vi "Find_Potentially_Stat_Dots_In_Dot-Matrix-1.vi"(4 "[IN] Count of event \"+1\"":i32, 5 "[IN] Dot matrix with \nstatuses after searching \nof unmoving dots":i16[][](array[numeric]), 6 "[IN] Possibly\nMoving (X,Y)":dbl[][](array[numeric]), 7 "Current # frame":i32, 8 "Y2":dbl, 9 "X2":dbl, 10 "Y1":dbl, 11 "X1":dbl) -> (1 "[OUT] Count of event \"+1\" 2":i32, 3 "[OUT] Dot matrix with \nstatuses after searching \nof unmoving dots":i16[][](array[numeric]))   [LabVIEW 2013]
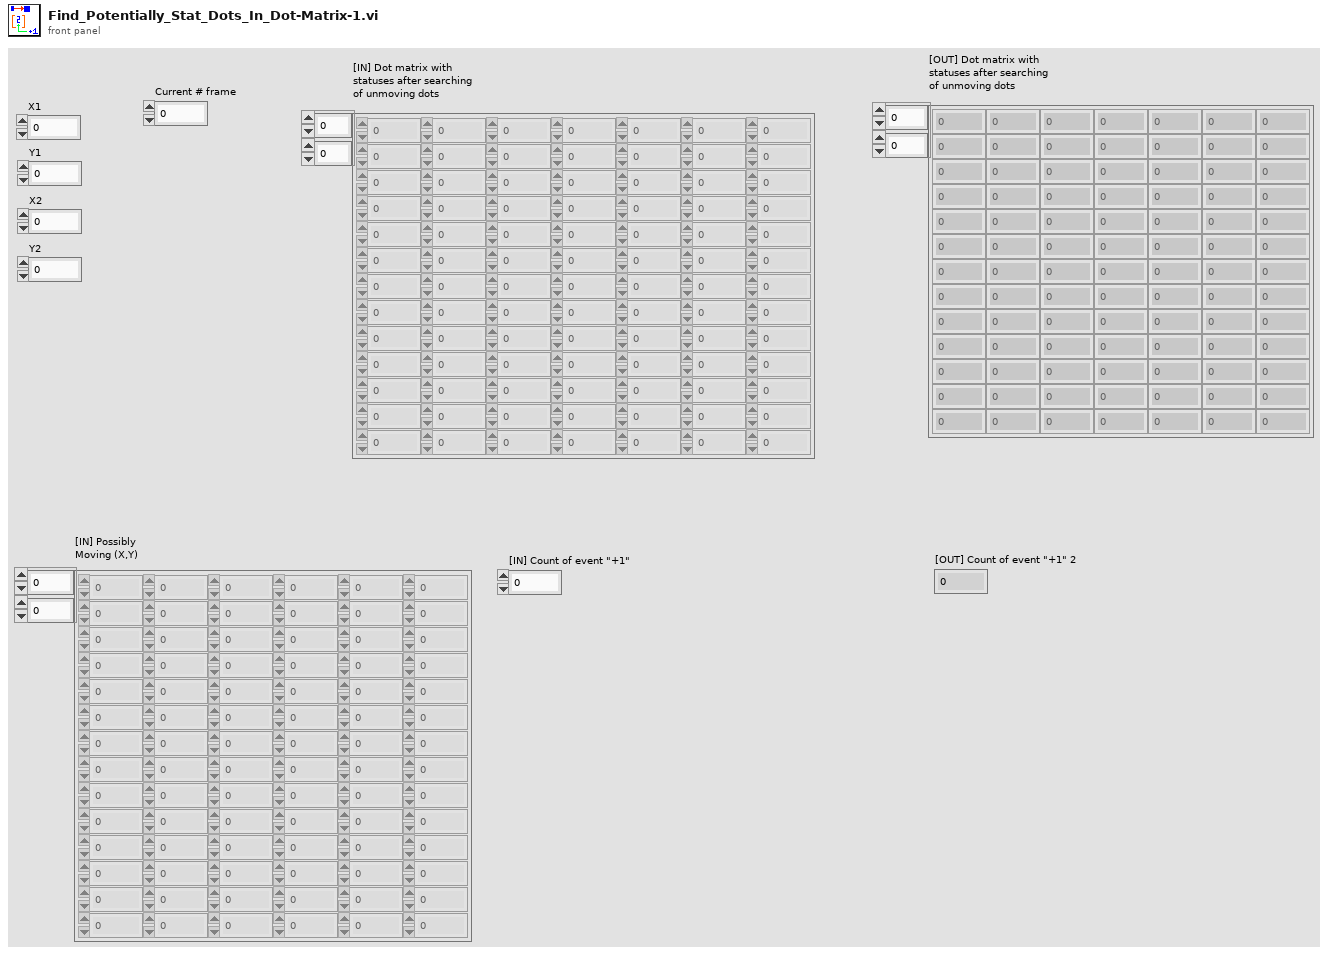
[diagram p1: front panel]
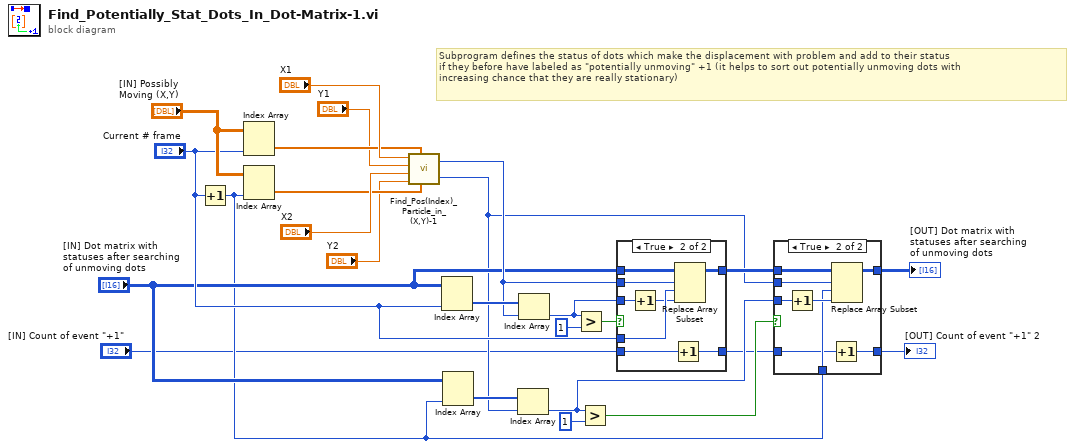
[diagram p0: block diagram]
diagram:
  # "Subprogram defines the status of dots which make the displacement with problem and add to their status\nif they before have labeled as \"potentially unmoving\" +1 (it helps to sort out potentially unmoving dots with\nincreasing chance that they are really stationary)"
  n1 = Increment(x="Current # frame") -> (x+1=w6:i32)
  n2 = Index Array(array="[IN] Possibly\nMoving (X,Y)", index (col)="Current # frame") -> (element=w23:dbl[])  [unwired: 1 in]
  n3 = Index Array(array="[IN] Possibly\nMoving (X,Y)", index (col)=w6) -> (element=w20:dbl[])  [unwired: 1 in]
  n4 = call "Find_Pos(Index)_Particle_in_(X,Y)-1.vi"("[X,Y] (n+1 Frame)"=w20, "[X,Y] (n Frame)"=w23, "Y2"="Y2", "X2"="X2", "Y1"="Y1", "X1"="X1") -> ("Index in (n+1) Frame"=w5:i32, "Index in (n) Frame"=w12:i32)
  n5 = Index Array(array="[IN] Dot matrix with \nstatuses after searching \nof unmoving dots", index (col)="Current # frame") -> (element=w18:i16[])  [unwired: 1 in]
  n6 = Index Array(array="[IN] Dot matrix with \nstatuses after searching \nof unmoving dots", index (col)=w6) -> (element=w17:i16[])  [unwired: 1 in]
  n7 = Index Array(array=w17, index=w5) -> (element=w8:i16)
  n8 = Index Array(array=w18, index=w12) -> (element=w14:i16)
  n9 = Greater?(x=w14, y=i16 1) -> (0:w15:bool)
  n10 = Greater?(x=w8, y=i16 1) -> (0:w7:bool)
  n11 = case shown="True" w15 {
    tunnel: w14 -> [_ w35]
    tunnel: "[IN] Dot matrix with \nstatuses after searching \nof unmoving dots" -> [w27 w34]
    tunnel: "Current # frame" -> [_ w33]
    tunnel: w12 -> [_ w32]
    tunnel: [w27 w30] -> w10
    tunnel: "[IN] Count of event \"+1\"" -> [w26 w29]
    tunnel: [w26 w28] -> w2
    frame False {
    }
    frame True {
      n12 = Increment(x=w35) -> (x+1=w31:i16)
      n13 = Increment(x=w29) -> (x+1=w28:i32)
      n14 = Replace Array Subset(array=w34, new element=w31, index (row)=w32, index (col)=w33) -> (w30:i16[][])
    }
  }
  n15 = case shown="True" w7 {
    tunnel: w8 -> [_ w45]
    tunnel: w10 -> [w37 w44]
    tunnel: w5 -> [_ w43]
    tunnel: [w37 w41] -> w4
    tunnel: w6 -> [_ w40]
    tunnel: w2 -> [w36 w39]
    tunnel: [w36 w38] -> w1
    frame False {
    }
    frame True {
      n16 = Increment(x=w45) -> (x+1=w42:i16)
      n17 = Increment(x=w39) -> (x+1=w38:i32)
      n18 = Replace Array Subset(array=w44, new element=w42, index (row)=w43, index (col)=w40) -> (w41:i16[][])
    }
  }
  "[OUT] Dot matrix with \nstatuses after searching \nof unmoving dots" <- w4
  "[OUT] Count of event \"+1\" 2" <- w1
